vi "Prueba 2 Elmin Mejia y Lester Roche.vi"() -> ()   [LabVIEW 2012]
panel:
  out "mayor a 40":bool
  out "contador>40":dbl
  out "temp promedio":dbl
  out "temp menor":dbl
  out "temp mayor":dbl
  out "temperatura":i32(slide) scale=0.0..60.0
  # "Se tiene que generar una temp entre 1-60, luego debera de encender un\nled cada vez que la temp sea mayor a 40 y debera de contarla.\nSe tiene que obtener el numero mayor y menor.\nLa temp promedio solo se obtiene de las temperaturas mayores a 30.\nHacerlo 5 veces, usar el ciclo for."
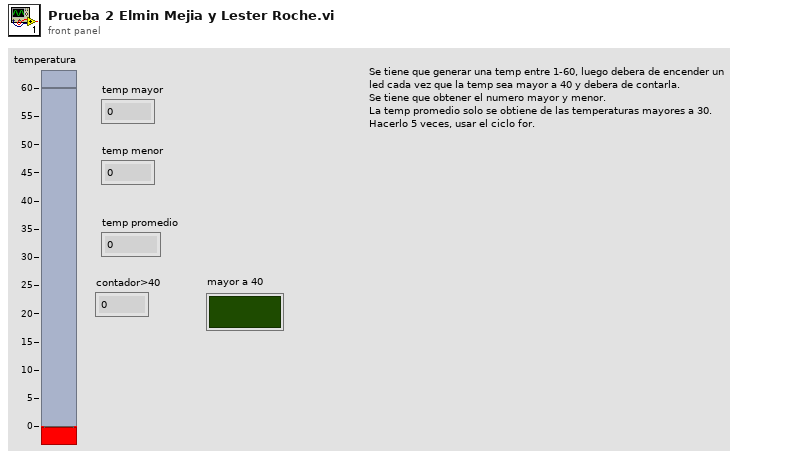
[diagram p1: front panel]
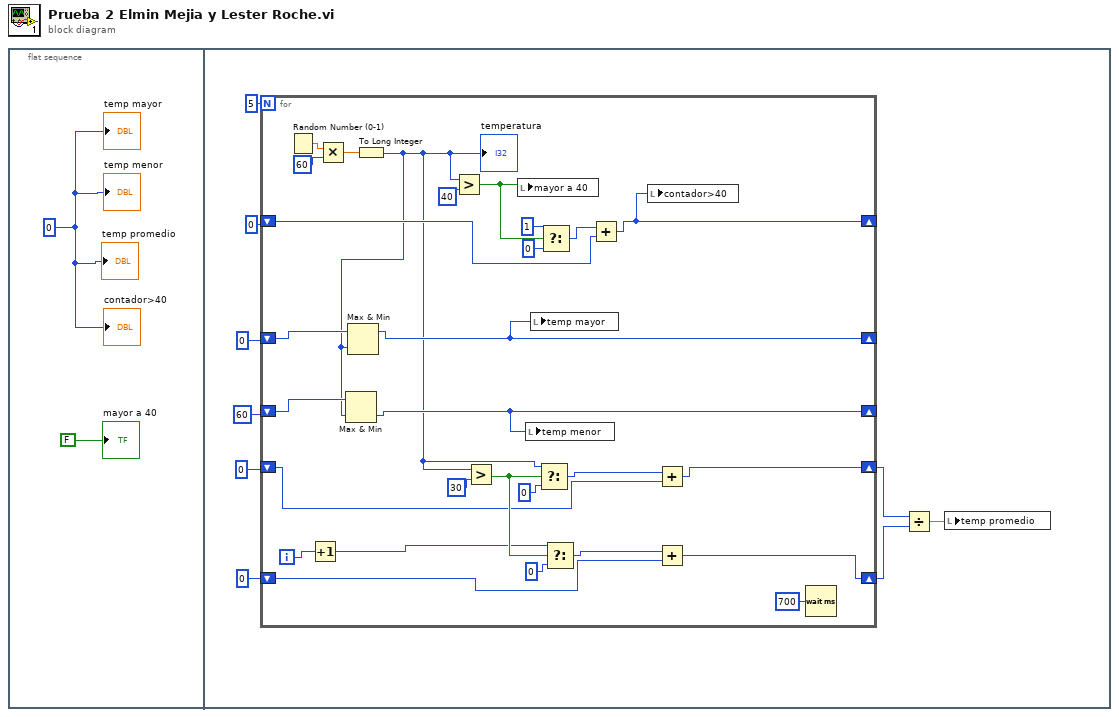
[diagram p0: block diagram]
diagram:
  n1 = flat-sequence {
    frame #0 {
      w2 = 0
      "temp mayor" <- w2
      "temp menor" <- w2
      "temp promedio" <- w2
      "contador>40" <- w2
      "mayor a 40" <- FALSE
    }
    frame #1 {
      n2 = for {
        N: 5 -> [_]
        shift-right: [w31] -> _
        shift-left: 0 -> [w32]
        shift-right: [w30] -> _
        shift-left: 60 -> [w28]
        shift-right: [w25] -> _
        shift-left: 0 -> [w26]
        shift-right: [w14] -> w5
        shift-left: 0 -> [w12]
        shift-right: [w13] -> w6
        shift-left: 0 -> [w16]
        i -> [w24]
        n3 = Random Number (0-1)() -> (number: 0 to 1=w37:dbl)
        n4 = Increment(x=w24) -> (x+1=w19:i32)
        n5 = Multiply(x=w37, y=60) -> (x*y=w39:dbl)
        n6 = To Long Integer(number=w39) -> (32bit integer=w22:i32)
        "temperatura" <- w22
        n7 = Max & Min(x=w28, y=w22) -> (min(x,y)=w30:i32)  [unwired: 1 out]
        n8 = Max & Min(x=w32, y=w22) -> (max(x,y)=w31:i32)  [unwired: 1 out]
        n9 = Greater?(x=w22, y=40) -> (0:w35:bool)
        n10 = Greater?(x=w22, y=30) -> (0:w20:bool)
        n11 = local write "mayor a 40"(w35) -> ()
        n12 = local write "temp menor"(w30) -> ()
        n13 = local write "temp mayor"(w31) -> ()
        n14 = Select(t=w22, s=w20, f=0) -> (s? t:f=w17:i32)
        n15 = Select(t=1, s=w35, f=0) -> (s? t:f=w27:i32)
        n16 = Select(t=w19, s=w20, f=0) -> (s? t:f=w15:i32)
        n17 = Add(x=w27, y=w26) -> (x+y=w25:i32)
        n18 = local write "contador>40"(w25) -> ()
        n19 = Add(x=w17, y=w16) -> (x+y=w13:i32)
        n20 = Add(x=w15, y=w12) -> (x+y=w14:i32)
        n21 = Wait (ms)(milliseconds to wait=700) -> ()  [unwired: 1 out]
      }
      n22 = Divide(x=w6, y=w5) -> (x/y=w4:dbl)
      n23 = local write "temp promedio"(w4) -> ()
    }
  }
